vi "Parse out Content.vi"(8 "error in (no error)":errorcluster, 11 "Response body":string) -> (0 "error out":errorcluster, 3 "Content":string)   [LabVIEW 2025, in "Battery Prompt.lvlib"]
doc: "Parses out the content from the GPT response without the use of JSON tools."
uses:
  Battery Prompt.lvlib
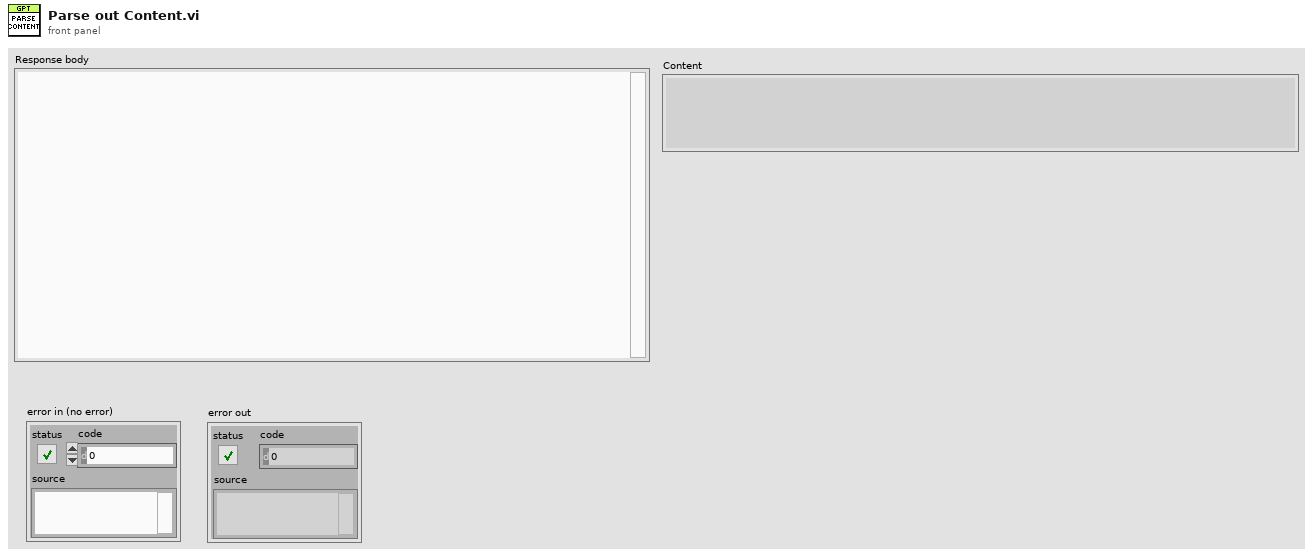
[diagram p1: front panel]
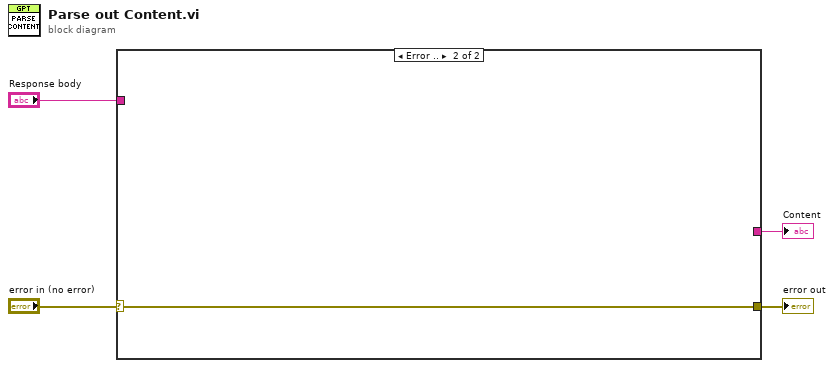
[diagram p0: block diagram]
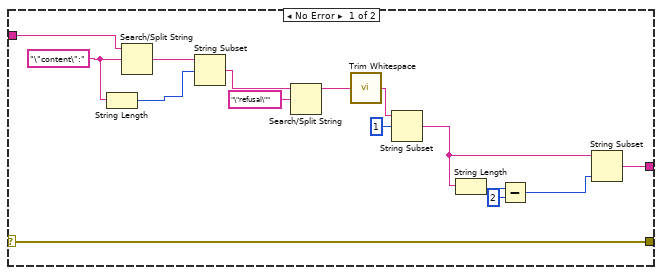
[diagram p2: hidden frame]
diagram:
  n1 = case shown="Error .." "error in (no error)" {
    selector: "error in (no error)" -> [w5 w20]
    tunnel: "Response body" -> [w19 _]
    tunnel: [w7 _] -> w3
    tunnel: [w5 w20] -> w1
    frame No Error {
      w17 = "\"content\":" ("search string/char (-)")
      n2 = String Length(string=w17) -> (length=w14:i32)
      n3 = Search/Split String(string=w19, search string/char (-)=w17) -> (match + rest of string=w18:string)  [unwired: 1 in, 2 out]
      n4 = String Subset(string=w18, offset (0)=w14) -> (substring=w15:string)  [unwired: 1 in]
      n5 = Search/Split String(string=w15, search string/char (-)="\"refusal\"") -> (substring before match=w13:string)  [unwired: 1 in, 2 out]
      n6 = call <vilib>:"Trim Whitespace.vi"("string"=w13) -> ("trimmed string"=w6:string)  [unwired: 1 in]
      n7 = String Subset(string=w6, offset (0)=1) -> (substring=w9:string)  [unwired: 1 in]
      n8 = String Length(string=w9) -> (length=w11:i32)
      n9 = Subtract(x=w11, y=2) -> (x-y=w8:i32)
      n10 = String Subset(string=w9, length (rest)=w8) -> (substring=w7:string)  [unwired: 1 in]
    }
    frame Error {
    }
  }
  "Content" <- w3
  "error out" <- w1
